vi "p8.15.vi"() -> ()   [LabVIEW 2020]
uses:
  <vilib>/vision/NI_Vision_Development_Module.lvlib
panel:
  out "Semillas Gaussiano":T1(plugin-control)
  in  "Kernel PB Gaussiano":sgl[][](array[numeric])=[[1.0, 2.0, 1.0, 0.0], [2.0, 4.0, 2.0, 0.0], [1.0, 2.0, 1.0, 0.0], [0.0, 0.0, 0.0, 1.0]] format="%.2f"
  out "Semillas":T1(plugin-control)
  out "Lenna boxcar":T1(plugin-control)
  in  "Kernel PB Boxcar":sgl[][](array[numeric])=[[1.0, 1.0, 1.0, 0.0], [1.0, 0.0, 1.0, 0.0], [1.0, 1.0, 1.0, 0.0], [0.0, 0.0, 0.0, 1.0]] format="%.2f"
  out "Lenna":T1(plugin-control)
  in  "Kernel Prewitt V":sgl[][](array[numeric])=[[-1.0, 0.0, 1.0, 0.0], [-1.0, 0.0, 1.0, 0.0], [-1.0, 0.0, 1.0, 0.0], [0.0, 0.0, 0.0, 1.0]] format="%.2f"
  out "Cruz Prewitt V":T1(plugin-control)
  out "cruz":T1(plugin-control)
  in  "Kernel Prewitt H":sgl[][](array[numeric])=[[-1.0, -1.0, -1.0, 0.0], [0.0, 0.0, 0.0, 0.0], [1.0, 1.0, 1.0, 0.0], [0.0, 0.0, 0.0, 1.0]] format="%.2f"
  out "Cruz Prewitt H":T1(plugin-control)
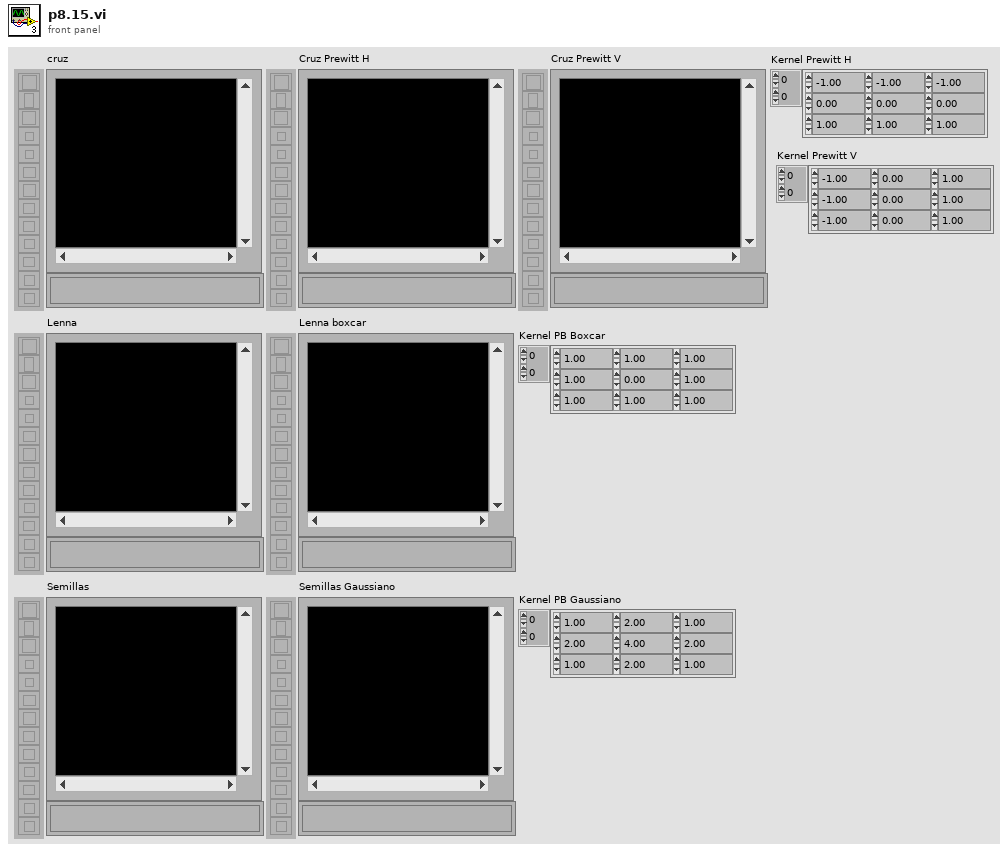
[diagram p1: front panel]
types:
  T1 = typedef "IMAQ Image.ctl" = refnum<image>
  T2 = typedef "Image Type" = u32
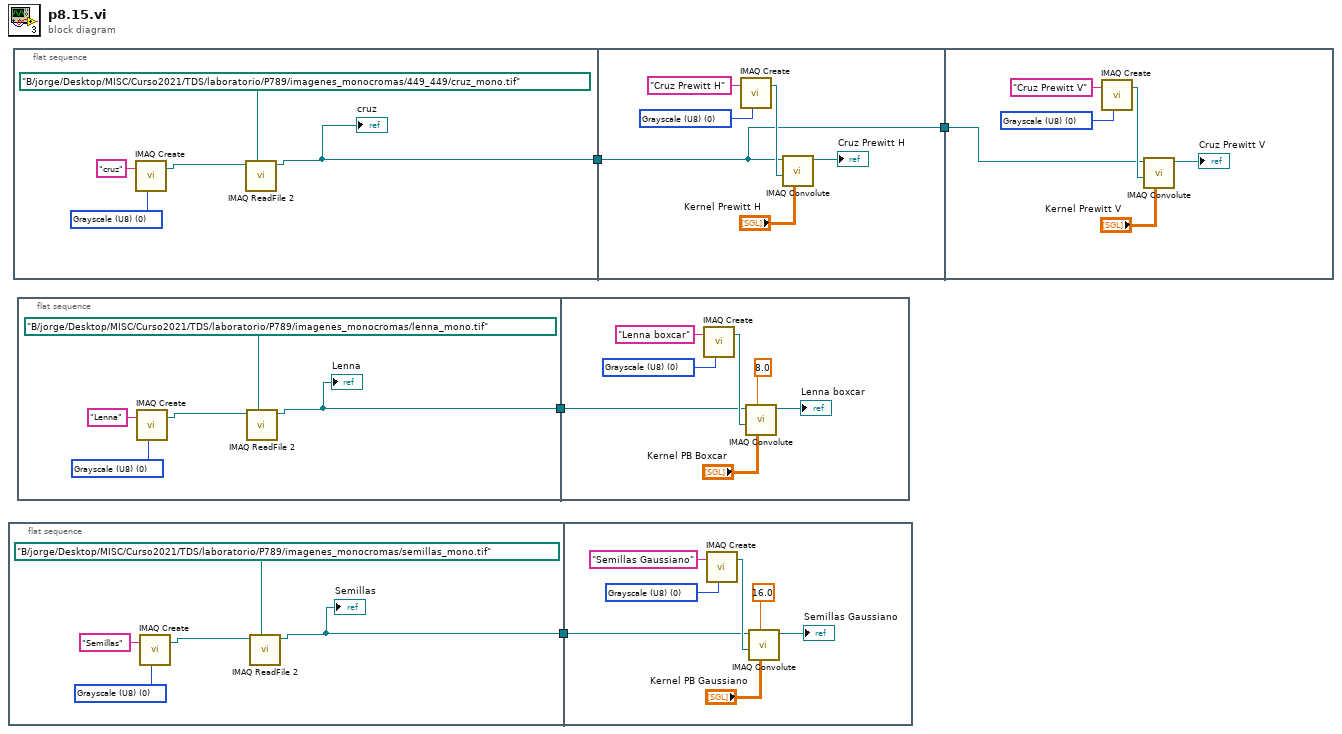
[diagram p0: block diagram]
diagram:
  n1 = flat-sequence {
    tunnel: [w6] -> w1
    tunnel: w1 -> [w11]
    frame #0 {
      w7 = T2 0 items=["Grayscale (U8)", "Grayscale (I16)", "Grayscale (SGL)", "Complex (CSG)", "RGB (U32)", "HSL (U32)", "RGB (U64)", "Grayscale (U16)"] ("Image Type")
      n2 = call "IMAQ Create"("Image Name"="Semillas", "Image Type"=w7) -> ("New Image"=w8:T1)  [unwired: 3 in, 1 out]
      n3 = call "IMAQ ReadFile 2"("File Path"=path "B:/jorge/Desktop/MISC/Curso2021/TDS/laboratorio/P789/imagenes_monocromas/semillas_mono.tif" ("Path cruz 2"), "Image"=w8) -> ("Image Out"=w6:T1)  [unwired: 5 in, 4 out]
      "Semillas" <- w6
    }
    frame #1 {
      w16 = T2 0 items=["Grayscale (U8)", "Grayscale (I16)", "Grayscale (SGL)", "Complex (CSG)", "RGB (U32)", "HSL (U32)", "RGB (U64)", "Grayscale (U16)"] ("Image Type")
      n4 = call "IMAQ Create"("Image Name"="Semillas Gaussiano", "Image Type"=w16) -> ("New Image"=w14:T1)  [unwired: 3 in, 1 out]
      n5 = call "IMAQ Convolute"("Kernel"="Kernel PB Gaussiano", "Divider (kernel sum)"=sgl 16.0, "Image Dst"=w14, "Image Src"=w11) -> ("Image Dst Out"=→"Semillas Gaussiano":T1)  [unwired: 6 in, 1 out]
    }
  }
  n6 = flat-sequence {
    tunnel: [w18] -> w4
    tunnel: w4 -> [w22]
    tunnel: [w22] -> w3
    tunnel: w3 -> [w28]
    frame #0 {
      w19 = T2 0 items=["Grayscale (U8)", "Grayscale (I16)", "Grayscale (SGL)", "Complex (CSG)", "RGB (U32)", "HSL (U32)", "RGB (U64)", "Grayscale (U16)"] ("Image Type")
      n7 = call "IMAQ Create"("Image Name"="cruz", "Image Type"=w19) -> ("New Image"=w20:T1)  [unwired: 3 in, 1 out]
      n8 = call "IMAQ ReadFile 2"("File Path"=path "B:/jorge/Desktop/MISC/Curso2021/TDS/laboratorio/P789/imagenes_monocromas/449_449/cruz_mono.tif" ("Path cruz"), "Image"=w20) -> ("Image Out"=w18:T1)  [unwired: 5 in, 4 out]
      "cruz" <- w18
    }
    frame #1 {
      w27 = T2 0 items=["Grayscale (U8)", "Grayscale (I16)", "Grayscale (SGL)", "Complex (CSG)", "RGB (U32)", "HSL (U32)", "RGB (U64)", "Grayscale (U16)"] ("Image Type")
      n9 = call "IMAQ Create"("Image Name"="Cruz Prewitt H", "Image Type"=w27) -> ("New Image"=w25:T1)  [unwired: 3 in, 1 out]
      n10 = call "IMAQ Convolute"("Kernel"="Kernel Prewitt H", "Image Dst"=w25, "Image Src"=w22) -> ("Image Dst Out"=→"Cruz Prewitt H":T1)  [unwired: 7 in, 1 out]
    }
    frame #2 {
      w33 = T2 0 items=["Grayscale (U8)", "Grayscale (I16)", "Grayscale (SGL)", "Complex (CSG)", "RGB (U32)", "HSL (U32)", "RGB (U64)", "Grayscale (U16)"] ("Image Type")
      n11 = call "IMAQ Create"("Image Name"="Cruz Prewitt V", "Image Type"=w33) -> ("New Image"=w31:T1)  [unwired: 3 in, 1 out]
      n12 = call "IMAQ Convolute"("Kernel"="Kernel Prewitt V", "Image Dst"=w31, "Image Src"=w28) -> ("Image Dst Out"=→"Cruz Prewitt V":T1)  [unwired: 7 in, 1 out]
    }
  }
  n13 = flat-sequence {
    tunnel: [w35] -> w2
    tunnel: w2 -> [w40]
    frame #0 {
      w36 = T2 0 items=["Grayscale (U8)", "Grayscale (I16)", "Grayscale (SGL)", "Complex (CSG)", "RGB (U32)", "HSL (U32)", "RGB (U64)", "Grayscale (U16)"] ("Image Type")
      n14 = call "IMAQ Create"("Image Name"="Lenna", "Image Type"=w36) -> ("New Image"=w37:T1)  [unwired: 3 in, 1 out]
      n15 = call "IMAQ ReadFile 2"("File Path"=path "B:/jorge/Desktop/MISC/Curso2021/TDS/laboratorio/P789/imagenes_monocromas/lenna_mono.tif" ("Path cruz 2"), "Image"=w37) -> ("Image Out"=w35:T1)  [unwired: 5 in, 4 out]
      "Lenna" <- w35
    }
    frame #1 {
      w45 = T2 0 items=["Grayscale (U8)", "Grayscale (I16)", "Grayscale (SGL)", "Complex (CSG)", "RGB (U32)", "HSL (U32)", "RGB (U64)", "Grayscale (U16)"] ("Image Type")
      n16 = call "IMAQ Create"("Image Name"="Lenna boxcar", "Image Type"=w45) -> ("New Image"=w43:T1)  [unwired: 3 in, 1 out]
      n17 = call "IMAQ Convolute"("Kernel"="Kernel PB Boxcar", "Divider (kernel sum)"=sgl 8.0, "Image Dst"=w43, "Image Src"=w40) -> ("Image Dst Out"=→"Lenna boxcar":T1)  [unwired: 6 in, 1 out]
    }
  }
